vi "SmartMotor Torque Monitor.vi"(8 "error in (no error)":errorcluster, 9 "Stop Motor Torque Monitor":bool, 11 "reference in":refnum<class "SmartMotor.lvclass">) -> (0 "error out":errorcluster, 3 "reference out":refnum<class "SmartMotor.lvclass">)   [LabVIEW 2017, in "SmartMotor.lvclass"]
uses:
  SmartMotor.lvclass
  <vilib>/Analysis/baseanly.llb/Mean (DBL).vi
  <vilib>/Analysis/NI_AALBase.lvlib
panel:
  out "Numeric 2":dbl
  out "Numeric":dbl
  out "Waveform Chart":cluster{i32, "mean":dbl}(graph)
  in  "Monitoring Duration (ms)":u32=20000
  # "This VI is called Asynchronously and will have one instance in memory\nfor each asynchronous call."
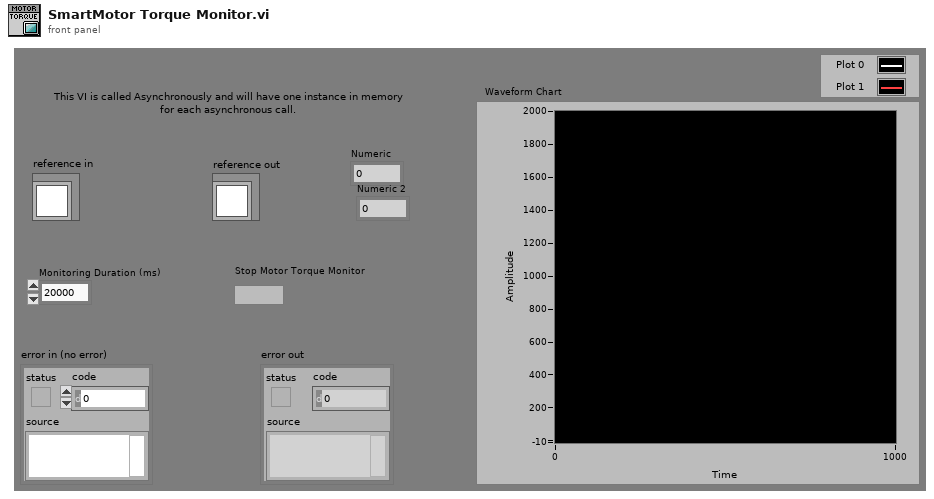
[diagram p1: front panel]
types:
  T1 = typedef "SmartMotor.lvclass/ObjectAttributes.ctl" = cluster{"SmartMotor Chain VISA Resource":refnum<visa-resource-name>, "SmartMotor Chain Address":i16, "Motor Absolute Position":i32, "Motor Relative Position":i32, "Motor Torque":i32, "Motor Voltage":i32, "Screwdriver Engaged":bool, "Screwdriver Torque Limit":i32, "Torque Monitor On/Off Status":bool, "Torque Monitor VI Reference":refnum<vi>, "Absolute Motor Torque (Filtered)":dbl, "SmartMotor Status":T2, "SmartMotor Error":T3}
  T2 = typedef "SmartMotor.lvclass/SmartMotor Status.ctl" = enum8{"Stopped", "Moving"}
  T3 = typedef "SmartMotor.lvclass/SmartMotor Error.ctl" = enum8{"None", "Read Error", "Low Voltage"}
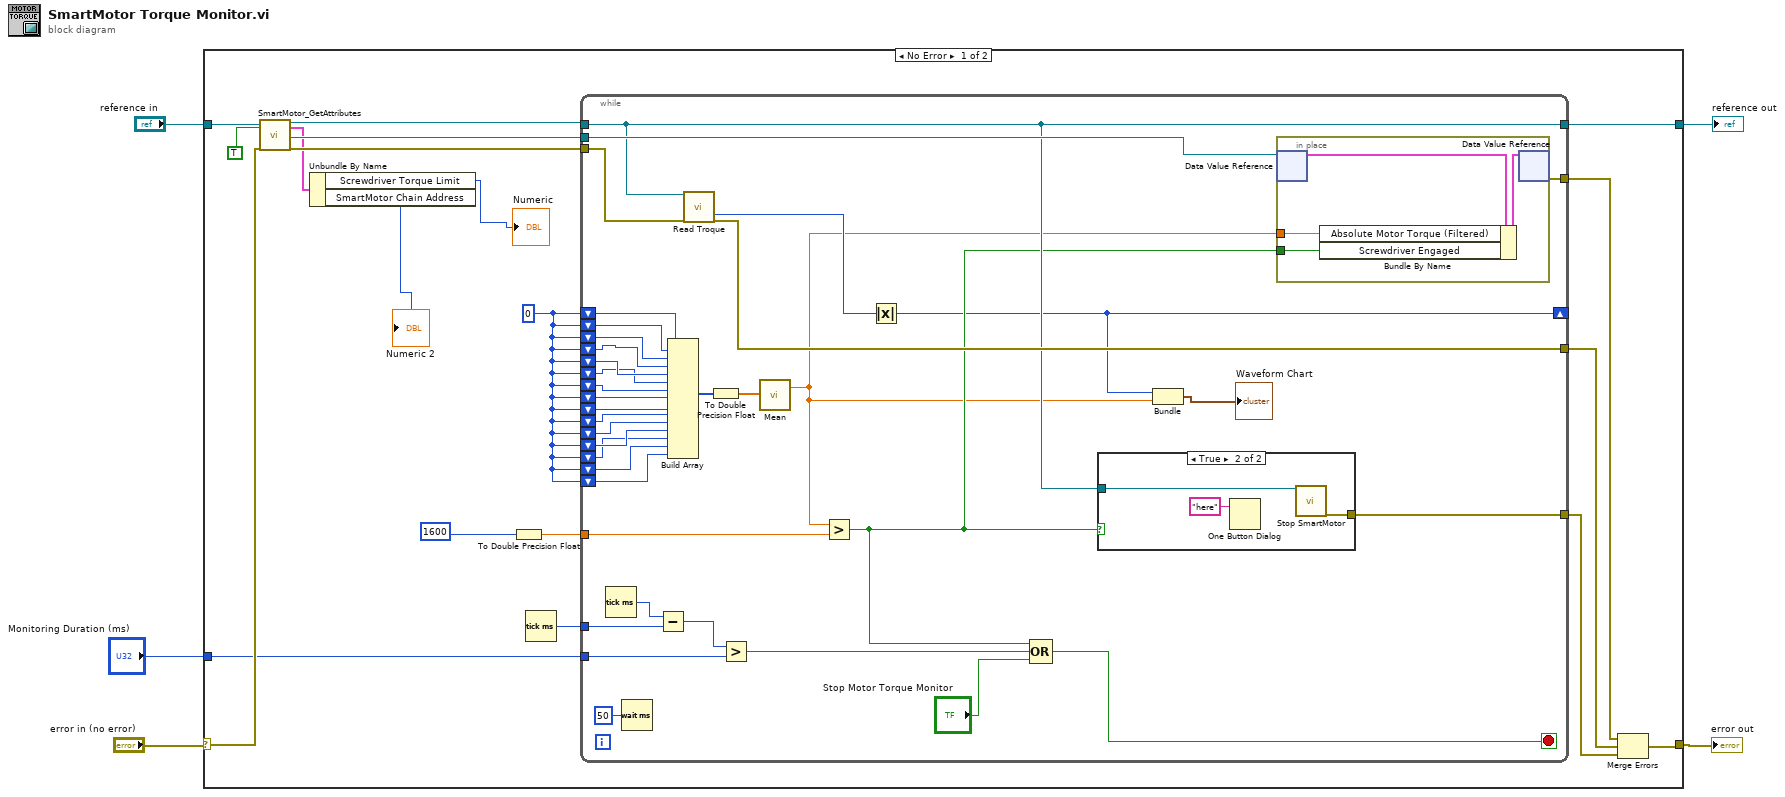
[diagram p0: block diagram]
diagram:
  n1 = case shown="No Error" "error in (no error)" {
    selector: "error in (no error)" -> [w18 w69]
    tunnel: "reference in" -> [w23 w70]
    tunnel: [w24 w70] -> w3
    tunnel: [w12 w69] -> w2
    tunnel: "Monitoring Duration (ms)" -> [w14 _]
    frame No Error {
      w17 = 0
      n2 = call "SmartMotor_GetAttributes.vi"("reference in"=w23, "OnlyGetDvrReference(False)"=TRUE, "error in (no error)"=w18) -> ("reference out"=w22:refnum<class "SmartMotor.lvclass">, "Data"=w16:T1, "DataRef"=w20:refnum<data-value>, "error out"=w19:errorcluster)  [unwired: 13 in]
      n3 = Unbundle By Name(w16) -> ("Screwdriver Torque Limit"=→"Numeric":i32, "SmartMotor Chain Address"=→"Numeric 2":i16)
      n4 = To Double Precision Float(number=1600) -> (double precision float=w15:dbl)
      n5 = Tick Count (ms)() -> (millisecond timer value=w13:u32)
      n6 = while {
        tunnel: w22 -> [w30]
        tunnel: [w30] -> w24
        tunnel: w20 -> [w61]
        tunnel: w19 -> [w60]
        shift-right: [w27] -> _
        shift-left: w17 -> [w55]
        shift-left: w17 -> [w54]
        shift-left: w17 -> [w53]
        shift-left: w17 -> [w52]
        shift-left: w17 -> [w51]
        shift-left: w17 -> [w50]
        shift-left: w17 -> [w49]
        shift-left: w17 -> [w48]
        shift-left: w17 -> [w47]
        shift-left: w17 -> [w46]
        shift-left: w17 -> [w45]
        shift-left: w17 -> [w44]
        shift-left: w17 -> [w43]
        shift-left: w17 -> [w42]
        shift-left: w17 -> [w41]
        tunnel: w15 -> [w40]
        tunnel: w14 -> [w36]
        tunnel: w13 -> [w35]
        tunnel: [w33] -> w11
        tunnel: [w32] -> w10
        tunnel: [w29] -> w9
        stop <- w31 stop-if-true
        n7 = Tick Count (ms)() -> (millisecond timer value=w38:u32)
        n8 = Wait (ms)(milliseconds to wait=u32 50) -> ()  [unwired: 1 out]
        n9 = Subtract(x=w38, y=w35) -> (x-y=w37:u32)
        n10 = Build Array(w55, w54, w53, w52, w51, w50, w49, w48, w47, w46, w45, w44, w43, w42, w41) -> (w56:i32[])
        n11 = call-dynamic "Read Troque.vi"("reference in"=w30, "error in (no error)"=w60) -> ("Motor Torque"=w58:i32, "error out"=w33:errorcluster)  [unwired: 15 in, 1 out]
        n12 = To Double Precision Float(number=w56) -> (double precision float=w57:dbl[])
        n13 = Greater?(x=w37, y=w36) -> (0:w34:bool)
        n14 = call-poly <vilib>:"Mean.vi"("X"=w57) -> ("mean"=w25:dbl)  [unwired: 1 out]
        n15 = Greater?(x=w25, y=w40) -> (0:w28:bool)
        n16 = Absolute Value(x=w58) -> (abs(x)=w27:i32)
        n17 = Compound Arithmetic op=OR(w28, w34, "Stop Motor Torque Monitor") -> (w31:bool)
        n18 = case shown="True" w28 {
          tunnel: w30 -> [_ w64]
          tunnel: [_ w63] -> w29
          frame False {
          }
          frame True {
            n19 = One Button Dialog(message="here") -> ()  [unwired: 1 in, 1 out]
            n20 = call-dynamic "Stop SmartMotor.vi"("reference in"=w64) -> ("error out"=w63:errorcluster)  [unwired: 17 in, 1 out]
          }
        }
        n21 = Bundle(w27, "mean"=w25) -> (→"Waveform Chart":cluster{i32, "mean":dbl})  [unwired: 1 in]
        n22 = in-place {
          in-place-border: w25 -> [w66]
          in-place-border: w28 -> [w65]
          n23 = in-place-dvr #1(w61) -> (w68:T1)  [unwired: 1 out]
          n24 = Bundle By Name(cluster=w68, "Absolute Motor Torque (Filtered)"=w66, "Screwdriver Engaged"=w65) -> (w67:T1)
          n25 = in-place-dvr #1(w67) -> (w32:errorcluster)  [unwired: 1 out]
        }
      }
      n26 = Merge Errors(w10, w11, w9) -> (w12:errorcluster)
    }
    frame Error {
    }
  }
  "error out" <- w2
  "reference out" <- w3
